vi "SPWB - About.vi"(5 "error in (no error)":errorcluster, 6 "ReInit All to Default?":bool, 7 "Application Name":string="GenUtil", 8 "Version #":string, 9 "State Queue":T1[](array[typedef])=["SC >>> Initialize"]) -> (19 "error out":errorcluster)   [LabVIEW 2022 SP3, in "SPWB.lvclass"]
uses:
  SPWB.lvclass
  API/Generic Utilities_class/utils/GenUtil State List.ctl
  <vilib>/Utility/sysdir.llb/System Directory Type.ctl
  <vilib>/Platform/browser.llb/Open URL in Default Browser (string).vi
  <vilib>/Platform/browser.llb/Open URL in Default Browser (path).vi
  API/Generic Utilities_class/Generic Utilities.lvclass
  <vilib>/addons/_AddQ/G#Object/G#Object.lvclass
panel:
  out "Title":string="Signal Processing WorkBench, "
  out "App Name:":string
  in  "SPWB Home":bool caption="If you find the SPWB software useful, please consider making a donation so we can continue developing and support this software.\nThanks in advance for your support and help!"
  in  "Exit":bool
  in  "Task":enum32{"Monitor", "Settings"}(tab)
  in  "AppData Folder":bool
  out "State History":string[](array[string])
  out "State Index":i32
  out "Exec Time":dbl
  in  "State 1":bool
  # "Ó Charette-AI-Group Inc. 2023"
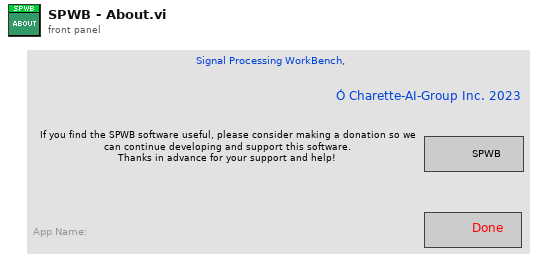
[diagram p1: front panel]
types:
  T1 = typedef "Generic Utilities.lvclass/GenUtil State List.ctl" = string
  T2 = enum32{"Invalid", "Standard", "Closed", "Hidden", "Minimized", "Maximized"}
  T3 = typedef "System Directory Type.ctl" = i32
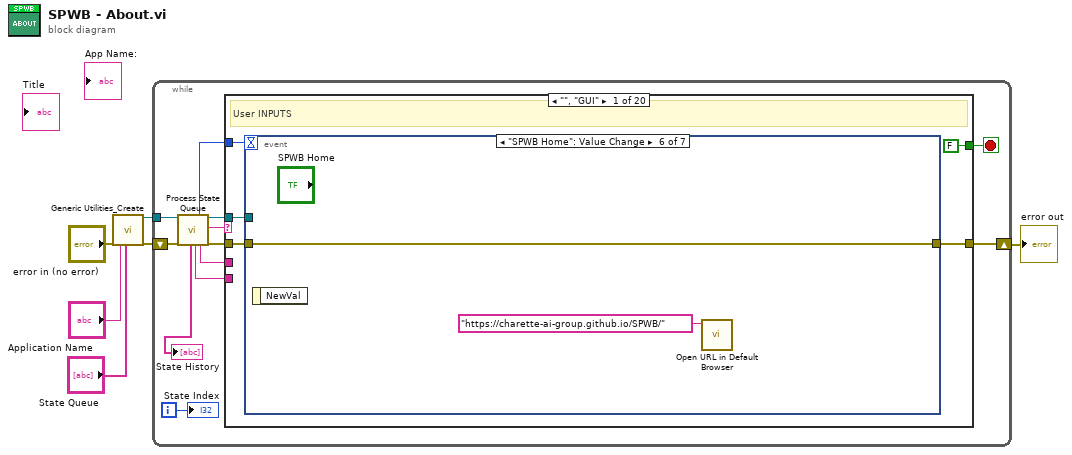
[diagram p0: block diagram]
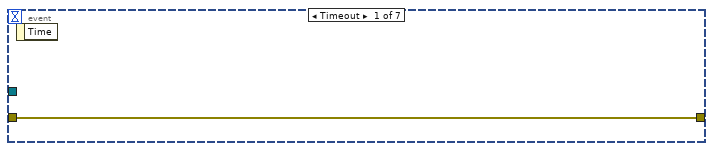
[diagram p2: hidden frame]
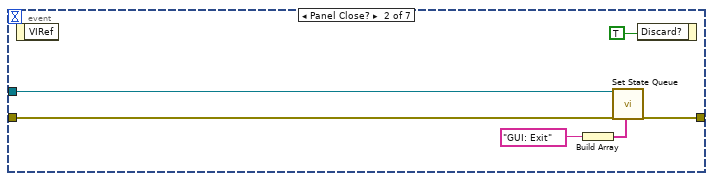
[diagram p3: hidden frame]
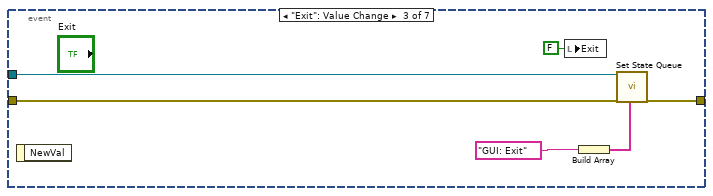
[diagram p4: hidden frame]
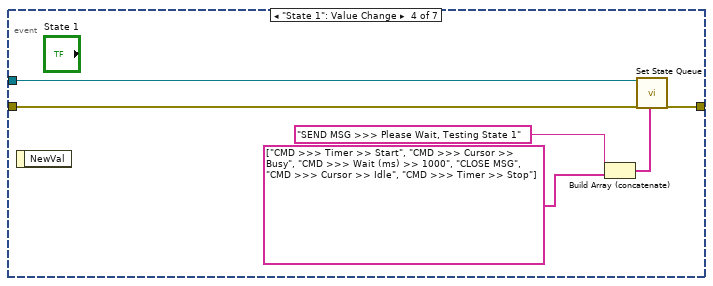
[diagram p5: hidden frame]
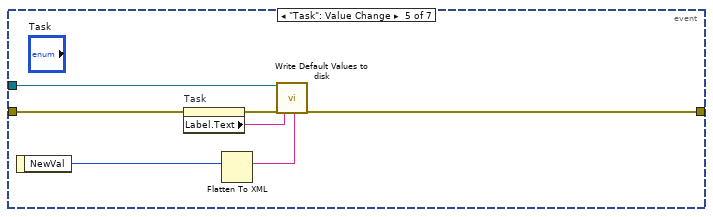
[diagram p6: hidden frame]
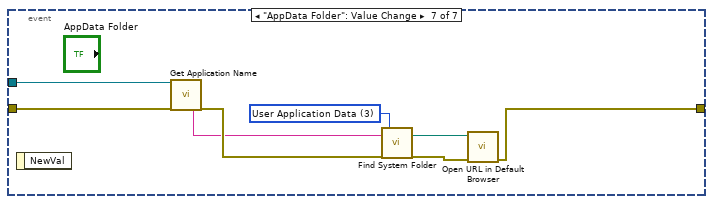
[diagram p7: hidden frame]
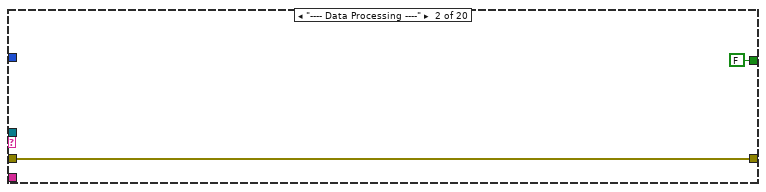
[diagram p8: hidden frame]
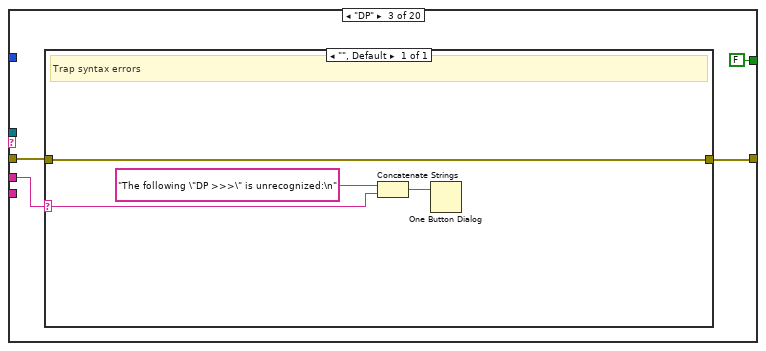
[diagram p9: hidden frame]
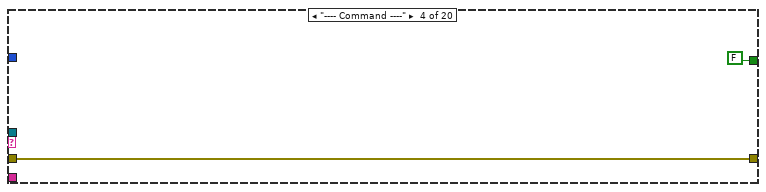
[diagram p10: hidden frame]
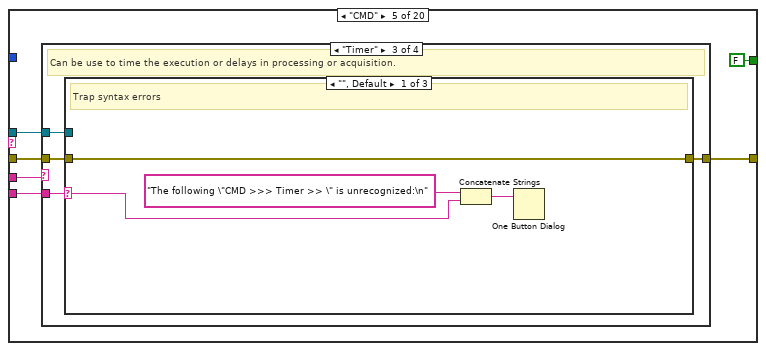
[diagram p11: hidden frame]
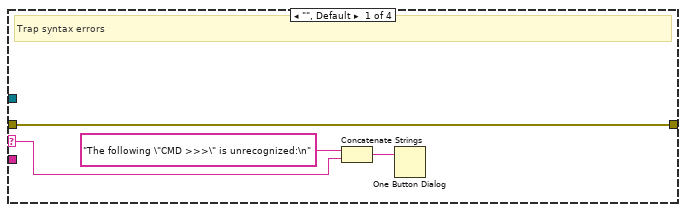
[diagram p12: hidden frame]
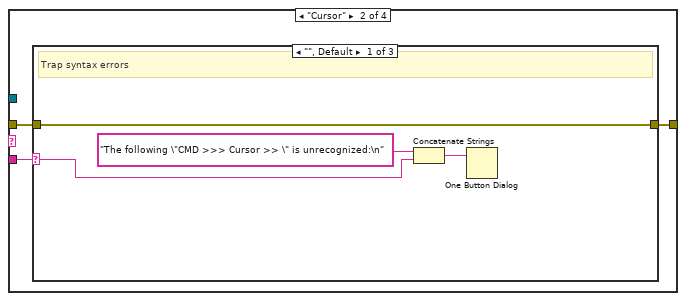
[diagram p13: hidden frame]
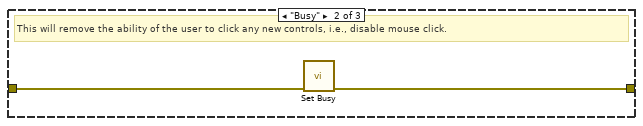
[diagram p14: hidden frame]
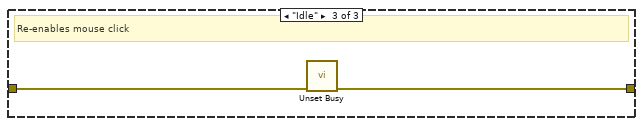
[diagram p15: hidden frame]
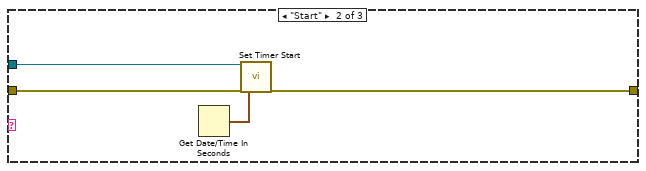
[diagram p16: hidden frame]
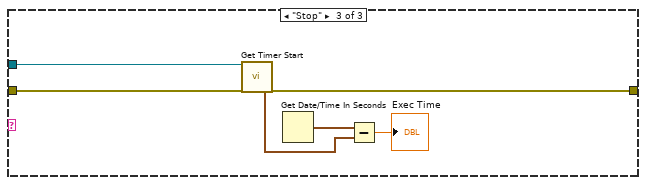
[diagram p17: hidden frame]
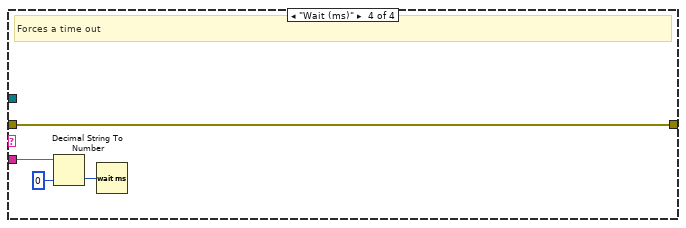
[diagram p18: hidden frame]
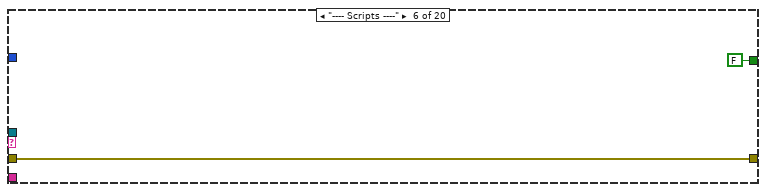
[diagram p19: hidden frame]
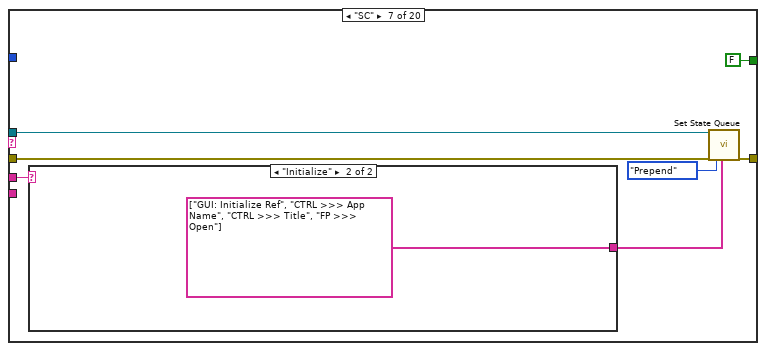
[diagram p20: hidden frame]
diagram:
  n1 = call "Generic Utilities_Create.vi"("error in (no error)"="error in (no error)", "Application Name"="Application Name", "State Queue"="State Queue") -> ("reference out"=w6:refnum<class "Generic Utilities.lvclass">, "error out"=w5:errorcluster)  [unwired: 15 in]
  n2 = while {
    shift-right: [w10] -> w1
    shift-left: w5 -> [w15]
    tunnel: w6 -> [w16]
    i -> [w17]
    stop <- w18 stop-if-true
    n3 = call "Process State Queue.vi"("reference in"=w16, "error in (no error)"=w15) -> ("State History"=→"State History":string[], "Additional Options"=w7:string, "Timeout"=w14:i32, "State Option"=w9:string, "reference out"=w13:refnum<class "Generic Utilities.lvclass">, "Current State"=w12:string, "error out"=w11:errorcluster)  [unwired: 10 in, 1 out]
    n4 = case shown="\"\", \"GUI\"" w12 {
      selector: w12 -> [_ _ _ _ _ _ _ _ _ _ _ _ _ _ _ _ w264 _ _ _]
      tunnel: w13 -> [w21 _ _ _ w72 _ w122 _ w133 w174 _ w205 w218 w253 w257 _ _ _ _ w274]
      tunnel: [FALSE FALSE FALSE FALSE FALSE FALSE FALSE FALSE FALSE FALSE FALSE FALSE TRUE FALSE FALSE FALSE FALSE FALSE FALSE TRUE] -> w18
      tunnel: w14 -> [w22 _ _ _ _ _ _ _ _ _ _ _ _ _ _ _ _ _ _ _]
      tunnel: w9 -> [_ _ w64 _ w76 _ w118 _ w134 w171 _ _ _ w250 _ _ _ _ _ _]
      tunnel: w11 -> [w20 w60 w63 w70 w74 w115 w121 w129 w131 w173 w194 w201 w215 w252 w258 w260 w262 w267 w270 w273]
      tunnel: [w19 w60 w62 w70 w75 w115 w120 w129 w132 w172 w194 w202 w214 w251 w256 w260 w262 errorcluster {"status"=FALSE, "code"=0, "source"=""} ("error out") w270 w272] -> w10
      tunnel: w7 -> [_ _ _ _ w73 _ _ _ _ _ _ _ _ _ _ _ _ _ _ _]
      frame "", "GUI" {
        # "User INPUTS"
        n5 = event shown="[5] \"SPWB Home\": Value Change" {
          selector: _ -> [_ _ _ _ _ _ _]
          dyn-events: _ -> [_ _ _ _ _ _ _]
          timeout: w22 -> [_ _ _ _ _ _ _]
          tunnel: w21 -> [_ w29 w35 w41 w48 _ w58]
          tunnel: w20 -> [w24 w28 w33 w40 w45 w50 w57]
          tunnel: [w24 w27 w34 w42 w43 w50 w52] -> w19
          event Timeout {
            n6 = event-data() -> ()  [unwired: 1 in, 1 out]
          }
          event Panel Close? {
            n7 = event-data() -> ()  [unwired: 1 in, 1 out]
            n8 = Build Array(T1 "GUI: Exit" ("State List")) -> (w26:T1[])
            n9 = call "Set State Queue.vi"("reference in"=w29, "error in (no error)"=w28, "State Queue"=w26) -> ("error out"=w27:errorcluster)  [unwired: 15 in, 1 out]
            n10 = event-data("Discard?"=TRUE) -> ()  [unwired: 1 in, 1 out]
          }
          event "Exit": Value Change {
            n11 = event-data() -> ()  [unwired: 1 in, 1 out]
            n12 = local write "Exit"(FALSE ("Exit")) -> ()
            n13 = Build Array(T1 "GUI: Exit" ("State List")) -> (w32:T1[])
            n14 = call "Set State Queue.vi"("reference in"=w35, "error in (no error)"=w33, "State Queue"=w32) -> ("error out"=w34:errorcluster)  [unwired: 15 in, 1 out]
          }
          event "State 1": Value Change {
            n15 = event-data() -> ()  [unwired: 1 in, 1 out]
            n16 = Build Array (concatenate)("SEND MSG >>> Please Wait, Testing State 1" ("String"), T1[] ["CMD >>> Timer >> Start", "CMD >>> Cursor >> Busy", "CMD >>> Wait (ms) >> 1000", "CLOSE MSG", "CMD >>> Cursor >> Idle", "CMD >>> Timer >> Stop"] ("State Queue OUT")) -> (w37:T1[])
            n17 = call "Set State Queue.vi"("reference in"=w41, "error in (no error)"=w40, "State Queue"=w37) -> ("error out"=w42:errorcluster)  [unwired: 15 in, 1 out]
          }
          event "Task": Value Change {
            n18 = event-data() -> ("NewVal"=w49:enum32{"Monitor", "Settings"})  [unwired: 1 in]
            n19 = property on="Task" class="TabCtl (strict)"(error in=w45) -> (error out=w44:errorcluster, "Label.Text"=w47:string)  [unwired: 1 in, 1 out]
            n20 = Flatten To XML(6:w49) -> (2:w46:string)
            n21 = call-dynamic "Write Default Values to disk.vi"("reference in"=w48, "error in (no error)"=w44, "Control Label"=w47, "Value (XML String)"=w46) -> ("error out"=w43:errorcluster)  [unwired: 14 in, 1 out]
          }
          event "SPWB Home": Value Change {
            n22 = event-data() -> ()  [unwired: 1 in, 1 out]
            n23 = call-poly <vilib>:"Open URL in Default Browser.vi"("URL"="https://charette-ai-group.github.io/SPWB/") -> ()  [unwired: 5 in, 2 out]
          }
          event "AppData Folder": Value Change {
            w59 = T3 3 items=["User Home"=0, "User Desktop"=1, "User Documents"=2, "User Application Data"=3, "User Preferences"=4, "User Temporary"=5, "Public Documents"=6, "Public Application Data"=7, "Public Preferences"=8, "Public Cache"=13, "System Core Libraries"=9, "System Installed Libraries"=10, "Application Files"=11, "Boot Volume Root"=12] ("system directory type")
            n24 = event-data() -> ()  [unwired: 1 in, 1 out]
            n25 = call "Get Application Name.vi"("reference in"=w58, "error in (no error)"=w57) -> ("Application Name"=w55:string, "error out"=w56:errorcluster)  [unwired: 15 in, 1 out]
            n26 = call "Find System Folder.vi"("Application Name"=w55, "error in (no error)"=w56, "system directory type"=w59) -> ("System Folder"=w54:path, "error out"=w53:errorcluster)  [unwired: 15 in]
            n27 = call-poly <vilib>:"Open URL in Default Browser.vi"("error in (no error)"=w53, "path"=w54) -> ("error out"=w52:errorcluster)  [unwired: 4 in, 1 out]
          }
        }
      }
      frame "---- Data Processing ----" {
      }
      frame "DP" {
        n28 = case shown="\"\", Default" w64 {
          selector: w64 -> [w67]
          tunnel: [w66] -> w62
          tunnel: w63 -> [w66]
          frame "", Default {
            # "Trap syntax errors"
            n29 = Concatenate Strings("The following \"DP >>>\" is unrecognized:\n", w67) -> (w68:string)
            n30 = One Button Dialog(message=w68) -> ()  [unwired: 1 in, 1 out]
          }
        }
      }
      frame "---- Command ----" {
      }
      frame "CMD" {
        n31 = case shown="\"Timer\"" w76 {
          selector: w76 -> [w79 _ _ _]
          tunnel: [w78 w83 w95 w114] -> w75
          tunnel: w74 -> [w78 w82 w94 w114]
          tunnel: w73 -> [_ w84 w96 w111]
          tunnel: w72 -> [_ _ w93 _]
          frame "", Default {
            # "Trap syntax errors"
            n32 = Concatenate Strings("The following \"CMD >>>\" is unrecognized:\n", w79) -> (w80:string)
            n33 = One Button Dialog(message=w80) -> ()  [unwired: 1 in, 1 out]
          }
          frame "Cursor" {
            n34 = case shown="\"\", Default" w84 {
              selector: w84 -> [w86 _ _]
              tunnel: [w85 w89 w91] -> w83
              tunnel: w82 -> [w85 w90 w92]
              frame "", Default {
                # "Trap syntax errors"
                n35 = Concatenate Strings("The following \"CMD >>> Cursor >> \" is unrecognized:\n", w86) -> (w87:string)
                n36 = One Button Dialog(message=w87) -> ()  [unwired: 1 in, 1 out]
              }
              frame "Busy" {
                # "This will remove the ability of the user to click any new controls, i.e., disable mouse click."
                n37 = call <vilib>:"Set Busy.vi"("error in (no error)"=w90) -> ("error out"=w89:errorcluster)  [unwired: 9 in, 1 out]
              }
              frame "Idle" {
                # "Re-enables mouse click"
                n38 = call <vilib>:"Unset Busy.vi"("error in (no error)"=w92) -> ("error out"=w91:errorcluster)  [unwired: 10 in]
              }
            }
          }
          frame "Timer" {
            # "Can be use to time the execution or delays in processing or acquisition."
            n39 = case shown="\"\", Default" w96 {
              selector: w96 -> [w98 _ _]
              tunnel: [w97 w102 w107] -> w95
              tunnel: w94 -> [w97 w103 w108]
              tunnel: w93 -> [_ w104 w109]
              frame "", Default {
                # "Trap syntax errors"
                n40 = Concatenate Strings("The following \"CMD >>> Timer >> \" is unrecognized:\n", w98) -> (w99:string)
                n41 = One Button Dialog(message=w99) -> ()  [unwired: 1 in, 1 out]
              }
              frame "Start" {
                n42 = Get Date/Time In Seconds() -> (seconds since 1Jan1904=w101:timestamp)
                n43 = call "Set Timer Start.vi"("reference in"=w104, "error in (no error)"=w103, "Timer Start"=w101) -> ("error out"=w102:errorcluster)  [unwired: 15 in, 1 out]
              }
              frame "Stop" {
                n44 = call "Get Timer Start.vi"("reference in"=w109, "error in (no error)"=w108) -> ("Timer Start"=w106:timestamp, "error out"=w107:errorcluster)  [unwired: 15 in, 1 out]
                n45 = Get Date/Time In Seconds() -> (seconds since 1Jan1904=w110:timestamp)
                n46 = Subtract(x=w110, y=w106) -> (x-y=→"Exec Time":dbl)
              }
            }
          }
          frame "Wait (ms)" {
            # "Forces a time out"
            n47 = Decimal String To Number(string=w111, default (0L)=u32 0 ("default (0 I32)")) -> (number=w112:u32)  [unwired: 1 in, 1 out]
            n48 = Wait (ms)(milliseconds to wait=w112) -> ()  [unwired: 1 out]
          }
        }
      }
      frame "---- Scripts ----" {
      }
      frame "SC" {
        n49 = case shown="\"Initialize\"" w118 {
          selector: w118 -> [w125 _]
          tunnel: [string[] [] ("State Queue OUT") string[] ["GUI: Initialize Ref", "CTRL >>> App Name", "CTRL >>> Title", "FP >>> Open"] ("State Queue OUT")] -> w119
          frame "False", Default {
            n50 = Concatenate Strings("The following \"Script\" is unrecognized:\n", w125) -> (w126:string)
            n51 = One Button Dialog(message=w126) -> ()  [unwired: 1 in, 1 out]
          }
          frame "Initialize" {
          }
        }
        n52 = call "Set State Queue.vi"("reference in"=w122, "error in (no error)"=w121, "State Queue Options"=enum16{"Replace", "Append", "Prepend"}."Prepend", "State Queue"=w119) -> ("error out"=w120:errorcluster)  [unwired: 14 in, 1 out]
      }
      frame "---- Front Panel Mgmt ----" {
      }
      frame "CTRL" {
        n53 = case shown="\"Title\"" w134 {
          selector: w134 -> [w138 _ _ _]
          tunnel: w133 -> [_ w146 w162 w170]
          tunnel: [w136 w141 w158 w163] -> w132
          tunnel: w131 -> [w136 w144 w161 w169]
          frame "unknown", Default {
            n54 = Concatenate Strings("The following control name is unrecognized:\n", w138) -> (w137:string)
            n55 = One Button Dialog(message=w137) -> ()  [unwired: 1 in, 1 out]
          }
          frame "Task Tab" {
            n56 = property on="Task" class="TabCtl (strict)"(error in=w144) -> (error out=w145:errorcluster, "Label.Text"=w143:string, "Value"=w148:enum32{"Monitor", "Settings"})  [unwired: 1 in, 1 out]
            n57 = call-dynamic "Read Default Values from Disk.vi"("reference in"=w146, "error in (no error)"=w145, "Control Label"=w143) -> ("Value (XML String)"=w140:string, "error out"=w142:errorcluster)  [unwired: 14 in, 1 out]
            n58 = case shown="\"\"" w140 {
              selector: w140 -> [w155 _]
              tunnel: [w150 w157] -> w149
              tunnel: w148 -> [w152 w157]
              tunnel: w142 -> [w153 w156]
              tunnel: [w153 w156] -> w147
              frame "anything", Default {
                n59 = Unflatten From XML(xml string=w155, type=w152, error in (no error)=w153) -> (value=w151:enum32{"Monitor", "Settings"}, error out=w154:errorcluster)
                n60 = Select(t=w152, s=w154, f=w151) -> (s? t:f=w150:enum32{"Monitor", "Settings"})
              }
              frame "" {
                # "Either the file was not found or there was some error"
              }
            }
            n61 = property on="Task" class="TabCtl (strict)"(error in=w147, "Value"=w149) -> (error out=w141:errorcluster)  [unwired: 1 in, 1 out]
          }
          frame "App Name" {
            n62 = call "Get Application Name.vi"("reference in"=w162, "error in (no error)"=w161) -> ("Application Name"=w159:string, "error out"=w160:errorcluster)  [unwired: 15 in, 1 out]
            n63 = property on="App Name:" class="Str"(error in=w160, "Value"=w159) -> (error out=w158:errorcluster)  [unwired: 1 in, 1 out]
          }
          frame "Title" {
            n64 = call "Get Version Number.vi"("reference in"=w170, "error in (no error)"=w169) -> ("Version #"=w166:string, "error out"=w168:errorcluster)  [unwired: 15 in, 1 out]
            n65 = property on="Title" class="Str"(error in=w168) -> (error out=w164:errorcluster, "Value"=w167:string)  [unwired: 1 in, 1 out]
            n66 = Concatenate Strings(w167, w166) -> (w165:string)
            n67 = property on="Title" class="Str"(error in=w164, "Value"=w165) -> (error out=w163:errorcluster)  [unwired: 1 in, 1 out]
          }
        }
      }
      frame "FP" {
        n68 = case shown="\"Open\"" w171 {
          selector: w171 -> [w176 _]
          tunnel: w174 -> [_ w184]
          tunnel: w173 -> [w177 w183]
          tunnel: [w177 w180] -> w172
          frame "unknown", Default {
            n69 = Concatenate Strings("The following FP Command name is unrecognized:\n", w176) -> (w178:string)
            n70 = One Button Dialog(message=w178) -> ()  [unwired: 1 in, 1 out]
          }
          frame "Open" {
            n71 = call-dynamic "Get VI Ref.vi"("reference in"=w184, "error in (no error)"=w183) -> ("GUI VI Ref"=w181:refnum<vi>, "error out"=w182:errorcluster)  [unwired: 14 in, 2 out]
            n72 = property class="VI"(reference=w181, error in=w182) -> (reference out=w186:refnum<vi>, error out=w187:errorcluster, "Front Panel.Open"=w185:bool)
            n73 = case shown="False" w185 {
              tunnel: [w190 w193] -> w180
              tunnel: w187 -> [w189 w193]
              tunnel: w186 -> [w188 _]
              frame False {
                n74 = invoke class="VI" method="FP.Open"(reference=w188, error in=w189, "Activate"=TRUE, "State"=T2."Standard") -> (error out=w190:errorcluster)  [unwired: 1 in, 4 out]
              }
              frame True {
              }
            }
          }
        }
      }
      frame "---- GUI Functions ----" {
      }
      frame "GUI: Initialize Ref" {
        n75 = control-ref of="GUI Reference"() -> (w200:refnum<vi>)
        n76 = call "Set VI Ref.vi"("reference in"=w205, "error in (no error)"=w201, "ReInit All to Default?"="ReInit All to Default?", "GUI VI Ref"=w200, "Version #"="Version #") -> ("reference out"=w204:refnum<class "Generic Utilities.lvclass">, "error out"=w199:errorcluster)  [unwired: 13 in]
        n77 = call "Set Close Panel (Yes or No).vi"("reference in"=w204, "error in (no error)"=w199) -> ("reference out"=w203:refnum<class "Generic Utilities.lvclass">, "error out"=w198:errorcluster)  [unwired: 16 in]
        n78 = call "Set Message Window Ref.vi"("reference in"=w203, "error in (no error)"=w198) -> ("error out"=w202:errorcluster)  [unwired: 16 in, 1 out]
      }
      frame "GUI: Exit" {
        n79 = call-dynamic "Get Message Window Ref.vi"("reference in"=w218, "error in (no error)"=w215) -> ("reference out"=w217:refnum<class "Generic Utilities.lvclass">, "Msg Win Ref"=w213:refnum<vi>, "error out"=w216:errorcluster)  [unwired: 15 in]
        n80 = call-dynamic "Get VI Ref.vi"("reference in"=w217, "error in (no error)"=w216) -> ("reference out"=w221:refnum<class "Generic Utilities.lvclass">, "GUI VI Ref"=w219:refnum<vi>, "error out"=w220:errorcluster)  [unwired: 14 in, 1 out]
        n81 = call-dynamic "Get Close Panel (Yes or No).vi"("reference in"=w221, "error in (no error)"=w220) -> ("Close Panel?"=w222:bool, "reference out"=w211:refnum<class "Generic Utilities.lvclass">, "error out"=w212:errorcluster)  [unwired: 15 in]
        n82 = call-dynamic "Get OBJ NOT RefNum.vi"("reference in"=w211, "error in (no error)"=w212) -> ("OBJ not a refnum?"=w210:bool, "reference out"=w209:refnum<class "Generic Utilities.lvclass">, "error out"=w208:errorcluster)  [unwired: 15 in]
        n83 = case shown="True" w210 {
          tunnel: [w227 w230] -> w207
          tunnel: w209 -> [_ w229]
          tunnel: w208 -> [w227 w228]
          frame False {
            # "The OBJ already exist, indicating this is a dialog box or sub-vi so do NOT destroy the original OBJ."
          }
          frame True {
            # "New OBJ was created, so it needs to be deleted."
            n84 = call-dynamic "Destroy.vi"("reference in"=w229, "error in (no error)"=w228) -> ("error out"=w231:errorcluster)  [unwired: 16 in, 1 out]
            n85 = disable-structure shown="Disabled" {
              disable-tunnel: w231 -> [w233 w234]
              disable-tunnel: [w232 w234] -> w230
              frame Disabled {
                # "Enable when NEEDED"
                n86 = call <vilib>:"GarbageCollector.vi"("error in (no error)"=w233) -> ("error out"=w232:errorcluster)  [unwired: 16 in, 2 out]
              }
              frame Enabled {
              }
            }
          }
        }
        n87 = Close Reference(reference=w213, error in (no error)=w207) -> (error out=w225:errorcluster)
        n88 = case shown="True" w222 {
          tunnel: w225 -> [w236 w240]
          tunnel: [w236 w239] -> w223
          tunnel: [w235 w238] -> w224
          tunnel: w219 -> [w235 w237]
          frame False {
          }
          frame True {
            n89 = property class="VI"(reference=w237, error in=w240) -> (reference out=w242:refnum<vi>, error out=w241:errorcluster, "Front Panel.Open"=w243:bool)
            n90 = case shown="True" w243 {
              tunnel: [w245 w249] -> w239
              tunnel: w241 -> [w245 w248]
              tunnel: w242 -> [w244 w247]
              tunnel: [w244 w246] -> w238
              frame False {
              }
              frame True {
                n91 = invoke class="VI" method="FP.Close"(reference=w247, error in=w248) -> (reference out=w246:refnum<vi>, error out=w249:errorcluster)  [unwired: 1 in, 1 out]
              }
            }
          }
        }
        n92 = Close Reference(reference=w224, error in (no error)=w223) -> (error out=w214:errorcluster)
      }
      frame "SEND MSG" {
        n93 = call-dynamic "Send Message.vi"("reference in"=w253, "error in (no error)"=w252, "Message (\"\" closes the window)"=w250) -> ("error out"=w251:errorcluster)  [unwired: 15 in, 1 out]
      }
      frame "CLOSE MSG" {
        n94 = call-dynamic "Send Message.vi"("reference in"=w257, "error in (no error)"=w258, "Message (\"\" closes the window)"="Close" ("Message")) -> ("error out"=w256:errorcluster)  [unwired: 15 in, 1 out]
      }
      frame "---- Miscelleneous ----" {
      }
      frame "unknown", Default {
        n95 = Concatenate Strings("The following state is unrecognized?\n", w264) -> (w263:string)
        n96 = One Button Dialog(message=w263) -> ()  [unwired: 1 in, 1 out]
      }
      frame "Error" {
        n97 = call <vilib>:"General Error Handler.vi"("error in (no error)"=w267) -> ()  [unwired: 10 in, 5 out]
      }
      frame "Next" {
        # "This is an empty case used so the queue does NOT stop if there is an empty string between two valid states!"
      }
      frame "Quit" {
        # "WARNING!, If the state machine crash, then it will also \"Quit\"??"
        # "This is the case used to simply exit when this GUI is used as a SubVI!"
        n98 = call-dynamic "Destroy.vi"("reference in"=w274, "error in (no error)"=w273) -> ("error out"=w272:errorcluster)  [unwired: 16 in, 1 out]
      }
    }
    "State Index" <- w17
  }
  "error out" <- w1
